vi "实例42 动态交互界面.vi"() -> ()   [LabVIEW 2014]
panel:
  in  "停止":bool
  out "字符串":string
  out "超速":bool
  out "速度":dbl(knob) scale=0.0..100.0
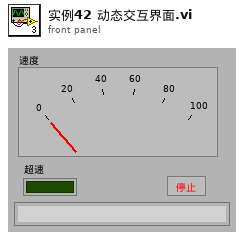
[diagram p1: front panel]
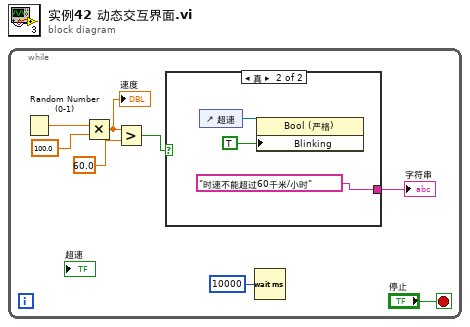
[diagram p0: block diagram]
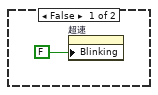
[diagram p2: hidden frame]
diagram:
  n1 = while {
    stop <- "停止" stop-if-true
    n2 = Random Number (0-1)() -> (number: 0 to 1=w8:dbl)
    n3 = Multiply(x=w8, y=100.0) -> (x*y=w4:dbl)
    "速度" <- w4
    n4 = Greater?(x=w4, y=60.0) -> (0:w2:bool)
    n5 = case shown="真" w2 {
      tunnel: [_ "时速不能超过60千米/小时" ("字符串")] -> w1
      frame False {
        n6 = property on="超速" class="Bool (严格)"("Blinking"=FALSE ("闪烁")) -> ()  [unwired: 2 in, 2 out]
      }
      frame True {
        n7 = control-ref of="超速"() -> (w12:refnum<vi>)
        n8 = property class="Bool (严格)"(reference=w12, "Blinking"=TRUE ("闪烁")) -> ()  [unwired: 1 in, 2 out]
      }
    }
    "字符串" <- w1
    n9 = Wait (ms)(milliseconds to wait=u32 10000 ("等待时间（毫秒）")) -> ()  [unwired: 1 out]
  }
